vi "TargetCalcGlobals.vi"() -> ()   [LabVIEW 2025]
panel:
  out "Target Loc Y":dbl
  out "Target Loc X":dbl
  out "Robot Odom Orient Rad":dbl
  out "Robot Odom Y":dbl
  out "Robot Odom X":dbl
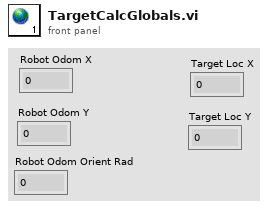
[diagram p1: front panel]
diagram:
